vi "Read Waveform.vi"   [LabVIEW 2011, in "Agilent DSO1000 Series.lvlib"]
doc: "Allows users to read one or more waveforms from the oscilloscope."
uses:
  <instrlib>/Agilent DSO1000 Series/Agilent DSO1000 Series.lvlib
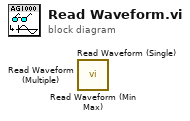
[diagram p0: block diagram]
diagram:
  n1 = call <instrlib>:"Read Waveform (Min Max).vi"() -> ()  [unwired: 8 in, 4 out]
  n2 = call <instrlib>:"Read Waveform (Single).vi"() -> ()  [unwired: 9 in, 3 out]
  n3 = call <instrlib>:"Read Waveform (Multiple).vi"() -> ()  [unwired: 9 in, 3 out]
